vi "GenericCommand.vi"(0 "Universal Robot.lvclass in":refnum<class "Universal Robot.lvclass">, 1 "command":string, 2 "data":string, 5 "error in (no error)":errorcluster) -> (14 "Universal Robot.lvclass out":refnum<class "Universal Robot.lvclass">, 15 "returnStatus":string, 16 "data out":string, 19 "error out":errorcluster)   [LabVIEW 2019, in "Universal Robot.lvclass"]
uses:
  Universal Robot.lvclass
  Universal Robot.lvclass/Universal Robot.ctl
  Client Interfaces/Dashboard Server/Dashboard Server.lvclass
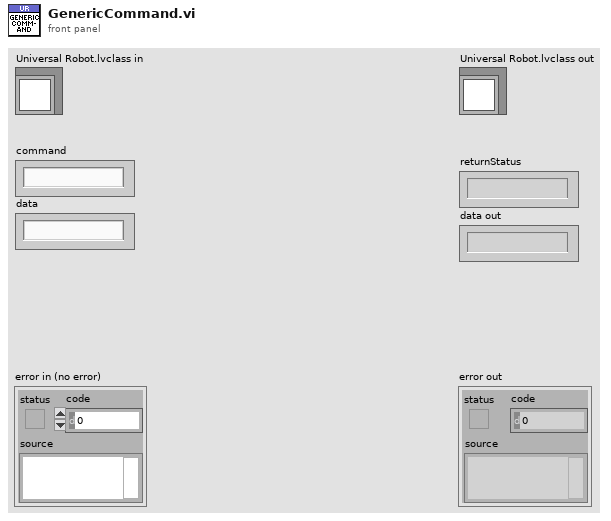
[diagram p1: front panel]
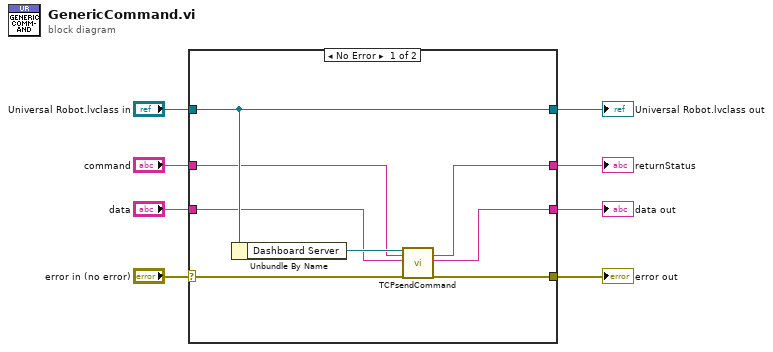
[diagram p0: block diagram]
diagram:
  n1 = case shown="No Error" "error in (no error)" {
    selector: "error in (no error)" -> [w15 w18]
    tunnel: [w14 w18] -> w7
    tunnel: "Universal Robot.lvclass in" -> [w16 w17]
    tunnel: [w16 w17] -> w5
    tunnel: "command" -> [w12 _]
    tunnel: "data" -> [w11 _]
    tunnel: [w10 _] -> w2
    tunnel: [w9 _] -> w1
    frame No Error {
      n2 = Unbundle By Name(w16) -> ("Dashboard Server"=w13:refnum<class "Dashboard Server.lvclass">)
      n3 = call-dynamic "TCPsendCommand.vi"("DashboardServer in"=w13, "command"=w12, "data"=w11, "error in (no error)"=w15) -> ("returnStatus"=w10:string, "data"=w9:string, "error out"=w14:errorcluster)  [unwired: 12 in, 1 out]
    }
    frame Error {
    }
  }
  "error out" <- w7
  "Universal Robot.lvclass out" <- w5
  "returnStatus" <- w2
  "data out" <- w1
